vi "Config Voltage After Close Outlet.vi"(8 "error in (no error)":errorcluster, 10 "Voltage":dbl, 11 "FPGA API in":refnum<class "FPGA API.lvclass">) -> (0 "error out":errorcluster, 3 "FPGA API out":refnum<class "FPGA API.lvclass">)   [LabVIEW 2019, in "FPGA API.lvclass"]
uses:
  FPGA API.lvclass
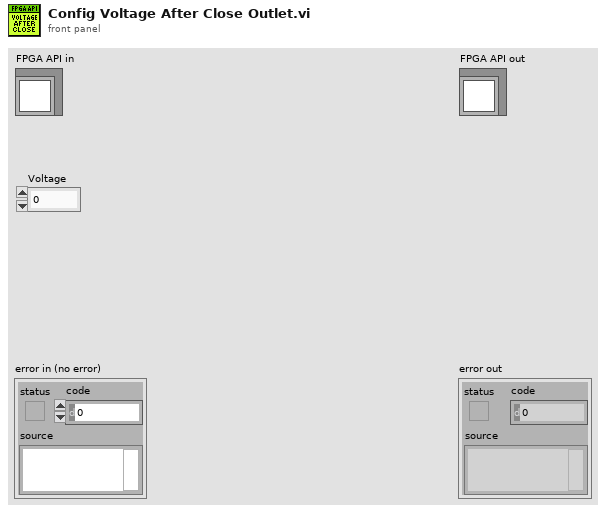
[diagram p1: front panel]
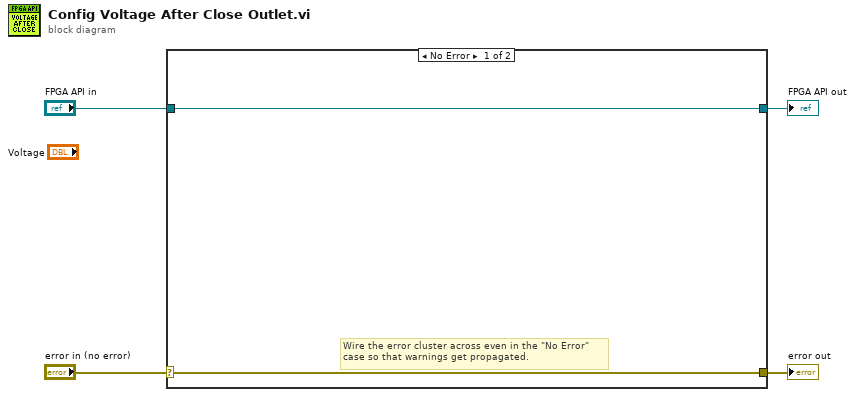
[diagram p0: block diagram]
diagram:
  n1 = case shown="No Error" "error in (no error)" {
    selector: "error in (no error)" -> [w5 w8]
    tunnel: [w5 w8] -> w3
    tunnel: [w6 w7] -> w1
    tunnel: "FPGA API in" -> [w6 w7]
    frame No Error {
      # "Wire the error cluster across even in the \"No Error\"\ncase so that warnings get propagated."
    }
    frame Error {
    }
  }
  "error out" <- w3
  "FPGA API out" <- w1
